vi "ZBX IO Arbiter.vi"(8 "response":T1, 10 "request 2":T2, 11 "request 1":T2) -> (0 "response 2":T1, 1 "response1":T1, 3 "request out":T2, 4 "protocol violation":u64)   [LabVIEW 2023]
doc: "Arbitrates requests for the DB IO. \nThis VI helps to ensure that requests to the DB IO are strictly serialized. It keeps track of the current request and sorts responses from the DB IO to the corresponding request. \nThe arbiter can be concatented with a other arbiters if more than two requests needs to be serialized."
uses:
  <instrlib>/niUSRP/Reference FPGA/ZBX Control/ZBX IO Arbiter States.ctl
  <instrlib>/_niInstr/Basic Elements/v1/FPGA/Private/Count Up U64.vi
  <instrlib>/niUSRP/Reference FPGA/ZBX Control/ZBX IO Request.ctl
  <instrlib>/niUSRP/Reference FPGA/ZBX Control/ZBX IO Response.ctl
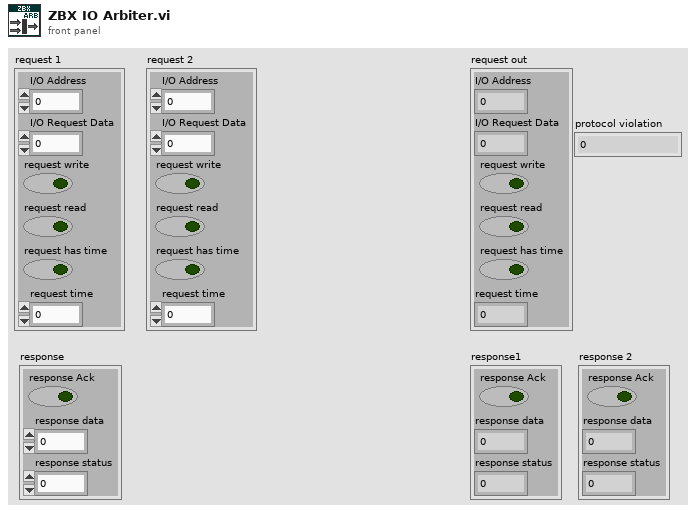
[diagram p1: front panel]
types:
  T1 = typedef "ZBX IO Response.ctl" = cluster{"response Ack":bool, "response data":u32, "response status":fxp<+,2,2>}
  T2 = typedef "ZBX IO Request.ctl" = cluster{"I/O Address":fxp<+,20,20>, "I/O Request Data":u32, "request write":bool, "request read":bool, "request has time":bool, "request time":u64}
  T3 = typedef "ZBX IO Arbiter States.ctl" = enum8{"Wait for Request", "Wait for Response"}
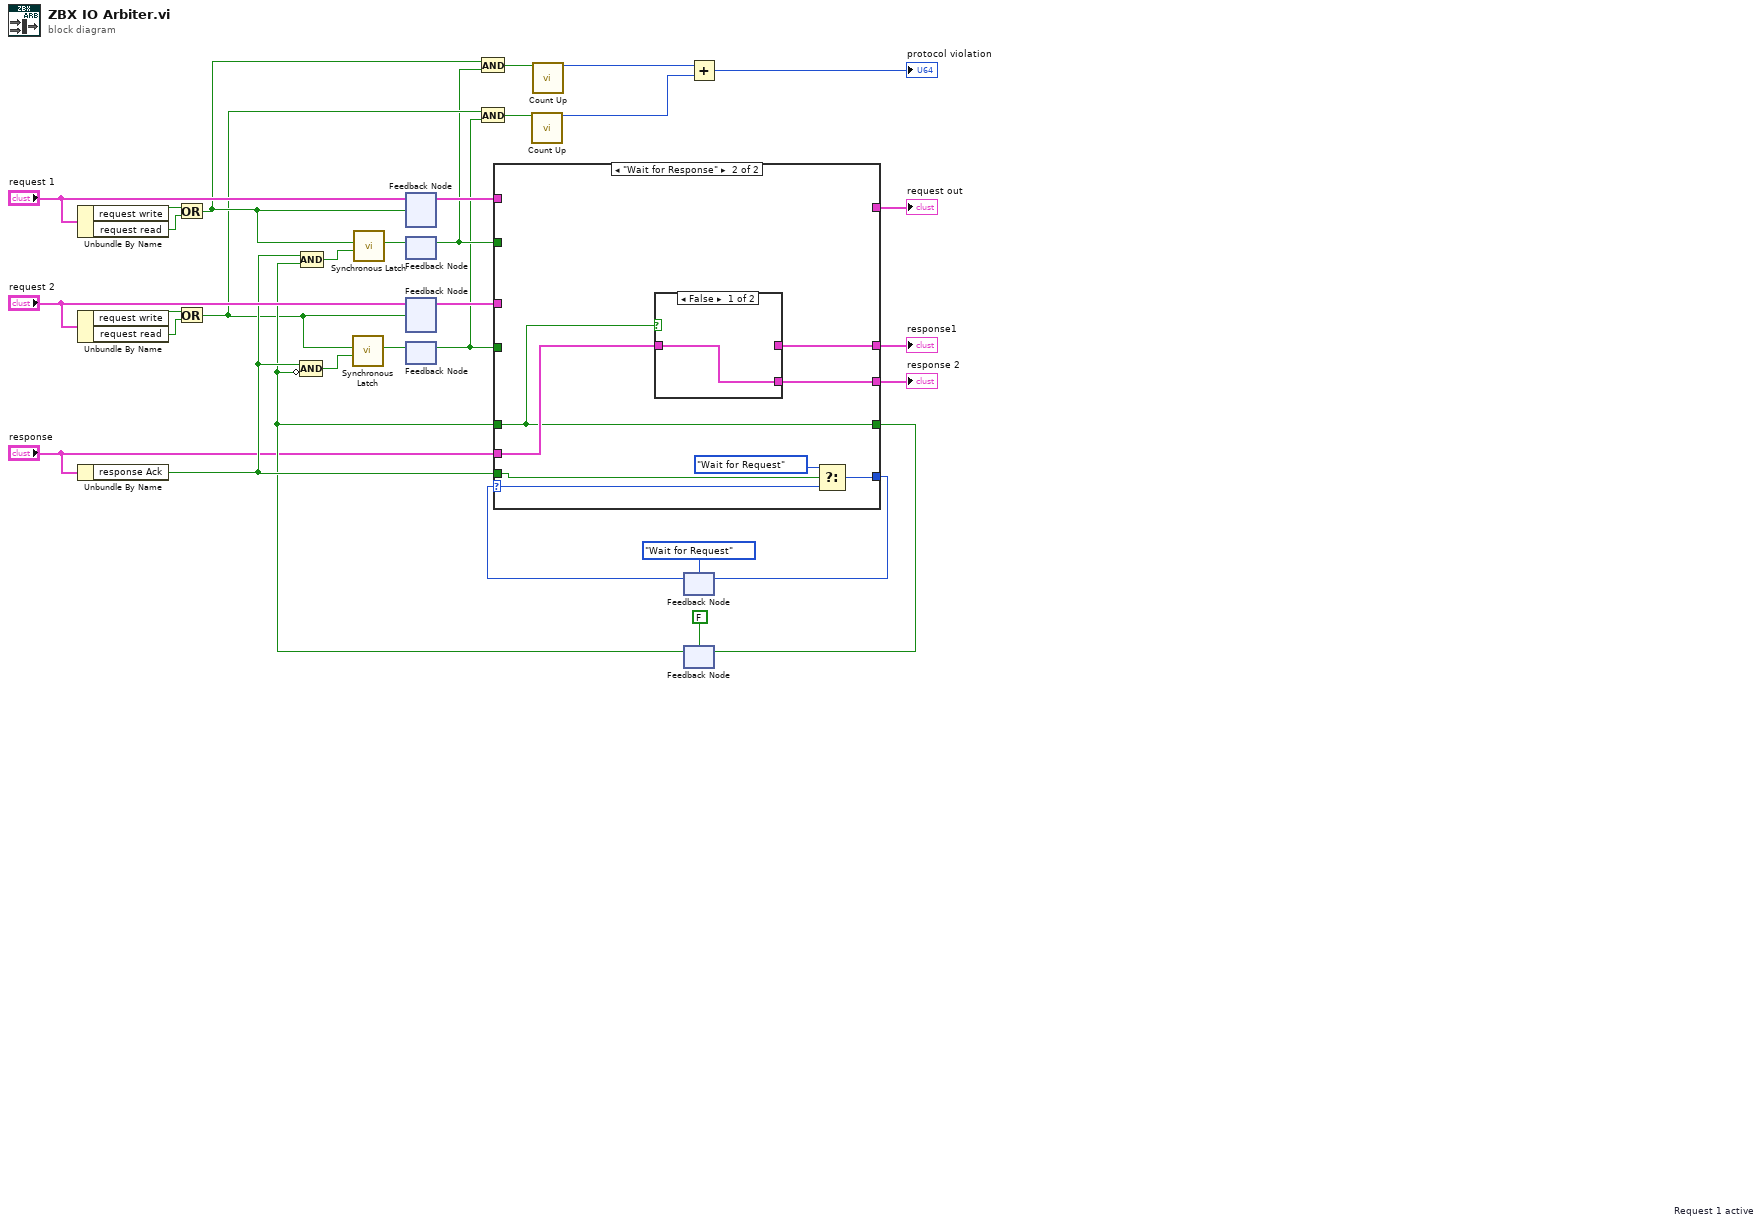
[diagram p0: block diagram]
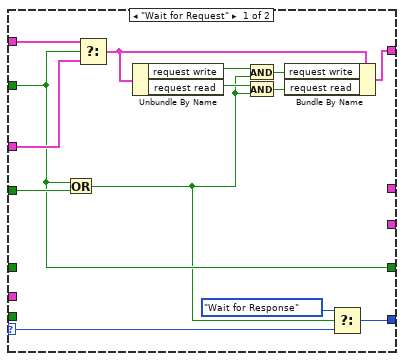
[diagram p2: hidden frame]
diagram:
  n1 = Unbundle By Name("request 1") -> ("request write"=w28:bool, "request read"=w29:bool)
  n2 = Unbundle By Name("request 2") -> ("request write"=w30:bool, "request read"=w31:bool)
  n3 = Unbundle By Name("response") -> ("response Ack"=w19:bool)
  n4 = Or(x=w28, y=w29) -> (x .or. y?=w13:bool)
  n5 = Or(x=w30, y=w31) -> (x .or. y?=w10:bool)
  n6 = feedback #1() -> (w25:T2)  [unwired: 1 in]
  n7 = feedback-in #1("request 1", w13) -> ()
  n8 = feedback #2() -> (w6:bool)  [unwired: 1 in]
  n9 = feedback #3() -> (w24:T2)  [unwired: 1 in]
  n10 = feedback-in #3("request 2", w10) -> ()
  n11 = feedback #4() -> (w5:bool)  [unwired: 1 in]
  n12 = And(x=w13, y=w6) -> (x .and. y?=w11:bool)
  n13 = And(x=w10, y=w5) -> (x .and. y?=w9:bool)
  n14 = call-poly <instrlib>:"Count Up.vi"("increment"=w9) -> ("count out"=w4:u64)  [unwired: 14 in]
  n15 = call-poly <instrlib>:"Count Up.vi"("increment"=w11) -> ("count out"=w8:u64)  [unwired: 14 in]
  n16 = feedback #5(ZBX_IO_Arbiter_States."Wait for Request") -> (w2:T3)
  n17 = feedback #6 "Request 1 active"(FALSE ("x .or. y?")) -> (w17:bool)
  n18 = Compound Arithmetic op=AND(w19, invert w17) -> (w18:bool)
  n19 = Compound Arithmetic op=AND(w19, w17) -> (w20:bool)
  n20 = call <instrlib>:"Synchronous Latch.vi"("clear"=w18, "set"=w10) -> ("out"=w7:bool)  [unwired: 9 in]
  n21 = call <instrlib>:"Synchronous Latch.vi"("clear"=w20, "set"=w13) -> ("out"=w12:bool)  [unwired: 9 in]
  n22 = feedback-in #2(w12) -> ()
  n23 = feedback-in #4(w7) -> ()
  n24 = case shown="\"Wait for Response\"" w2 {
    selector: w2 -> [w45 w51]
    tunnel: w6 -> [w42 _]
    tunnel: w5 -> [w46 _]
    tunnel: w25 -> [w44 _]
    tunnel: w24 -> [w43 _]
    tunnel: [w38 _] -> w21
    tunnel: "response" -> [_ w54]
    tunnel: w17 -> [_ w49]
    tunnel: [w42 w49] -> w22
    tunnel: [_ w53] -> w15
    tunnel: [_ w52] -> w14
    tunnel: w19 -> [_ w50]
    tunnel: [w41 w47] -> w1
    frame "Wait for Request" {
      n25 = Or(x=w42, y=w46) -> (x .or. y?=w33:bool)
      n26 = Select(t=w44, s=w42, f=w43) -> (s? t:f=w39:T2)
      n27 = Unbundle By Name(w39) -> ("request write"=w36:bool, "request read"=w34:bool)
      n28 = And(x=w36, y=w33) -> (x .and. y?=w37:bool)
      n29 = And(x=w34, y=w33) -> (x .and. y?=w35:bool)
      n30 = Bundle By Name(cluster=w39, "request write"=w37, "request read"=w35) -> (w38:T2)
      n31 = Select(t=ZBX_IO_Arbiter_States."Wait for Response", s=w33, f=w45) -> (s? t:f=w41:T3)
    }
    frame "Wait for Response" {
      n32 = case shown="False" w49 {
        tunnel: w54 -> [w55 w56]
        tunnel: [_ w56] -> w53
        tunnel: [w55 _] -> w52
        frame False {
        }
        frame True {
        }
      }
      n33 = Select(t=ZBX_IO_Arbiter_States."Wait for Request", s=w50, f=w51) -> (s? t:f=w47:T3)
    }
  }
  "request out" <- w21
  "response1" <- w15
  "response 2" <- w14
  n34 = feedback-in #5(w1) -> ()
  n35 = feedback-in #6(w22) -> ()
  n36 = Add(x=w8, y=w4) -> (x+y=→"protocol violation":u64)
